vi "Frequency Response (Real-Im).vi"(0 "scaled signal X [EUx]":dbl[](array[numeric]) format="%.2f", 1 "scaled signal Y [EUy]":dbl[](array[numeric]) format="%.2f", 2 "sampling frequency [Hz]":dbl=10000.0 format="%.2f", 4 "channel X info":T2={"sensor sensitivity [mV/EU]"=1000.0, "engineering units"=1, "dB reference [EU]"=1.0, "custom label"="EU", "weighting filter"=0, "pregain [dB]"=0.0} {"pregain [dB]" format="%.2f"; "weighting filter" items=["Linear", "A-weighting", "B-weighting", "C-weighting", "ITU-R 468-4", "Dolby", "CCITT", "C-message"]; "dB reference [EU]" format="%^.1e"; "engineering units" items=["custom..."=0, "V"=1, "A"=21, "Pa"=2, "N"=20, "g"=3, "m/s^2"=4, "m/s"=5, "m"=6, "mm/s"=12, "mm"=13, "microns/s"=14, "microns"=15, "in/s^2"=7, "in/s"=8, "in"=9, "mils/s"=10, "mils"=11, "rad/s^2"=16, "rad/s"=17, "rad"=18, "strain"=19]; "sensor sensitivity [mV/EU]" format="%.2f"}, 5 "channel Y info":T2={"sensor sensitivity [mV/EU]"=1000.0, "engineering units"=1, "dB reference [EU]"=1.0, "custom label"="EU", "weighting filter"=0, "pregain [dB]"=0.0} {"pregain [dB]" format="%.2f"; "weighting filter" items=["Linear", "A-weighting", "B-weighting", "C-weighting", "ITU-R 468-4", "Dolby", "CCITT", "C-message"]; "dB reference [EU]" format="%^.1e"; "engineering units" items=["custom..."=0, "V"=1, "A"=21, "Pa"=2, "N"=20, "g"=3, "m/s^2"=4, "m/s"=5, "m"=6, "mm/s"=12, "mm"=13, "microns/s"=14, "microns"=15, "in/s^2"=7, "in/s"=8, "in"=9, "mils/s"=10, "mils"=11, "rad/s^2"=16, "rad/s"=17, "rad"=18, "strain"=19]; "sensor sensitivity [mV/EU]" format="%.2f"}, 6 "window":T6=1 items=["None"=0, "Hanning"=1, "Hamming"=2, "Blackman-Harris"=3, "Exact Blackman"=4, "Blackman"=5, "Flat Top"=6, "4 Term B-Harris "=7, "7 Term B-Harris"=8, "Low Sidelobe"=9, "Force - Exponential"=10, "Blackman Nuttall"=11, "Triangle"=30, "Bartlett-Hanning"=31, "Bohman"=32, "Parzen"=33, "Welch"=34, "Kaiser"=60, "Dolph-Chebyshev"=61, "Gaussian"=62], 7 "reset averaging (T)":bool=TRUE, 8 "force/exp settings":T5={"force window [%]"=50.0, "exponential window [%]"=10.0} {"exponential window [%]" min=0.0 max=100.0 format="%.2f"; "force window [%]" min=0.0 max=100.0 format="%.2f"}, 9 "averaging parameters":T1={"averaging mode"=enum."RMS averaging", "weighting mode"=enum."Linear", "number of averages"=10} {"number of averages" min=1}, 10 "FRF mode":enum16{"H1", "H2", "H3"}(ring)) -> (12 "df [Hz]":dbl format="%.2f", 13 "window constants":cluster{"eq noise BW":dbl, "coherent gain":dbl} {"coherent gain" format="%.2f"; "eq noise BW" format="%.2f"}, 14 "real part [EUy/EUx rms]":dbl[](array[numeric]) format="%.2f", 15 "imaginary part [EUy/EUx rms]":dbl[](array[numeric]) format="%.2f", 16 "unit label":string, 17 "coherence":dbl[](array[numeric]) format="%.2f", 18 "averages completed":dbl format="%.2f", 19 "error out":errorcluster)   [LabVIEW 2017]
doc: "Computes the frequency response and the coherence based on the input signals. Typically, X signal is the stimulus, and Y signal is the response of the system. Results are returned as real and imaginary parts.\nFrequency response is typically an averaged measurement. Each block of data corresponds to a single FFT block and must be passed individually to this VI. The first time this VI is called, reset averaging must be TRUE (default value), to start a new averaging process. For subsequent calls, reset averaging must be FALSE to continue the averaging process. Averages completed returns the number of averages completed so far.\nAveraging parameters specifies how the averaging is performed. This includes the averaging mode (no averaging, vector averaging, or RMS averaging), the weighting mode (linear or exponential), and the number of averages (used only if the weighting mode is exponential)."
uses:
  <vilib>/addons/_NISVFA/_Shared subVIs/Controls/svc_Window [Dual FFT].ctl
  <vilib>/addons/Sound and Vibration/compatibility/Controls/svl_Channel Info.ctl
  <vilib>/addons/Sound and Vibration/compatibility/Controls/svl_Engineering Units Text Ring.ctl
  <vilib>/addons/Sound and Vibration/compatibility/Controls/svl_Weighting Filter Text Ring.ctl
  <vilib>/Analysis/4window.llb/Force Window (DBL).vi
  <vilib>/Analysis/4window.llb/Exponential Window (DBL).vi
  <vilib>/Analysis/2dsp.llb/Real FFT.vi
  <vilib>/Analysis/2dsp.llb/Power Spectrum (DBL).vi
  <vilib>/Analysis/2dsp.llb/Cross Power (DBL).vi
  <vilib>/Analysis/0measdsp.llb/Scaled Time Domain Window (DBL).vi
  <vilib>/Analysis/NI_AALPro.lvlib
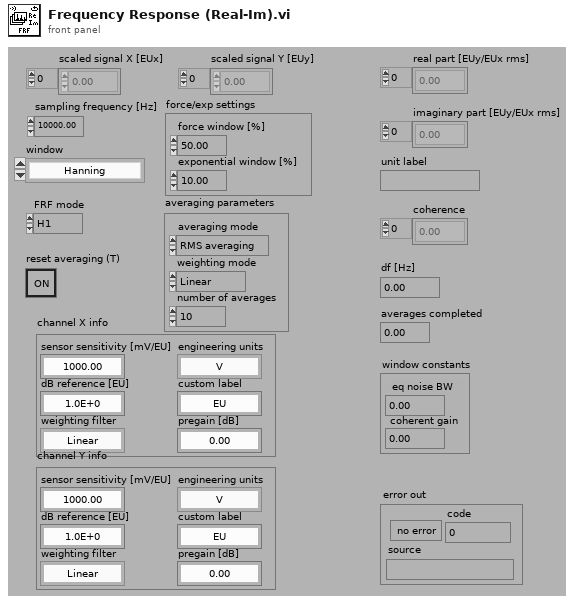
[diagram p1: front panel]
types:
  T1 = cluster{"averaging mode":enum16{"No averaging", "Vector averaging", "RMS averaging"}, "weighting mode":enum16{"Linear", "Exponential"}, "number of averages":u32}
  T2 = typedef "svl_Channel Info.ctl" = cluster{"sensor sensitivity [mV/EU]":dbl, "engineering units":T3, "dB reference [EU]":dbl, "custom label":string, "weighting filter":T4, "pregain [dB]":dbl}
  T3 = typedef "svl_Engineering Units Text Ring.ctl" = u16
  T4 = typedef "svl_Weighting Filter Text Ring.ctl" = u16
  T5 = cluster{"force window [%]":dbl, "exponential window [%]":dbl}
  T6 = typedef "svc_Window [Dual FFT].ctl" = u32
  T7 = enum16{"No averaging", "Vector averaging", "RMS averaging"}
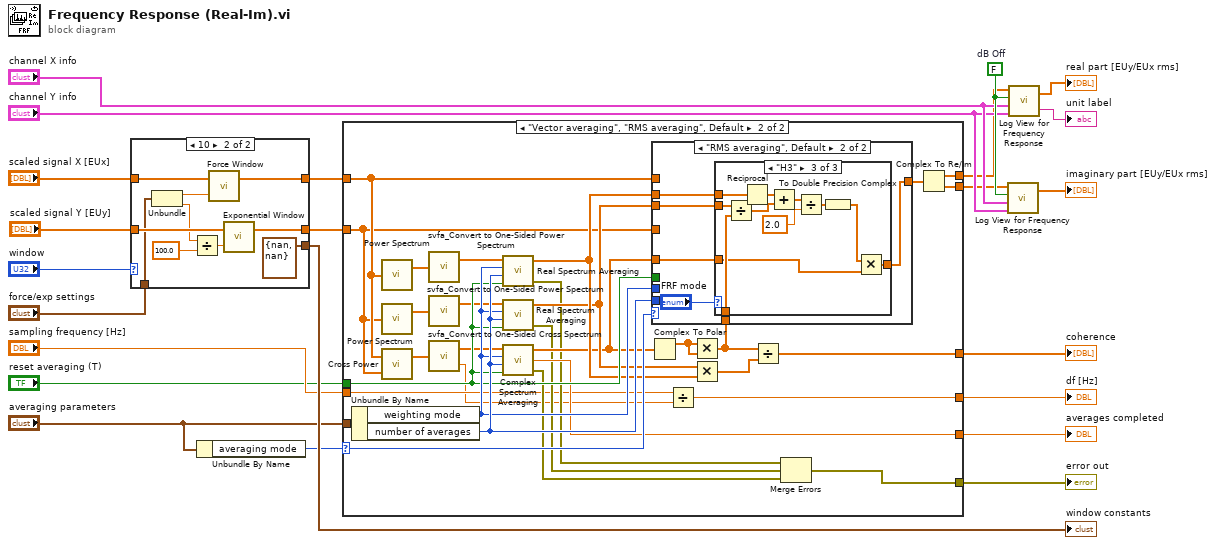
[diagram p0: block diagram]
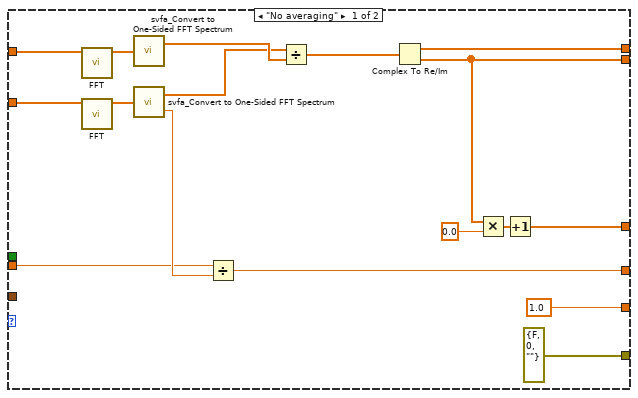
[diagram p2: hidden frame]
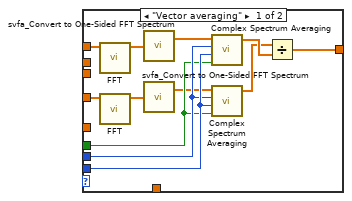
[diagram p3: hidden frame]
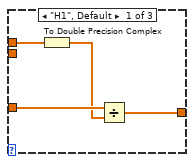
[diagram p4: hidden frame]
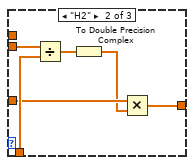
[diagram p5: hidden frame]
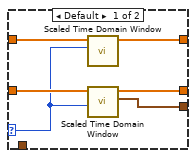
[diagram p6: hidden frame]
diagram:
  w10 = FALSE  # dB Off
  n1 = case shown="10" "window" {
    selector: "window" -> [w24 _]
    tunnel: "scaled signal X [EUx]" -> [w29 w39]
    tunnel: "scaled signal Y [EUy]" -> [w28 w38]
    tunnel: "force/exp settings" -> [_ w34]
    tunnel: [w27 w36] -> w19
    tunnel: [w26 w35] -> w18
    tunnel: [w25 cluster{"eq noise BW":dbl, "coherent gain":dbl} {"eq noise BW"=nan, "coherent gain"=nan} ("window constants")] -> w20
    frame Default {
      n2 = call-poly <vilib>:"Scaled Time Domain Window.vi"("window"=w24, "X"=w29) -> ("Windowed X"=w27:dbl[])  [unwired: 7 in, 2 out]
      n3 = call-poly <vilib>:"Scaled Time Domain Window.vi"("window"=w24, "X"=w28) -> ("window properties"=w25:cluster{"eq noise BW":dbl, "coherent gain":dbl}, "Windowed X"=w26:dbl[])  [unwired: 7 in, 1 out]
    }
    frame 10 {
      n4 = Unbundle(w34) -> ("force window [%]"=w33:dbl, "exponential window [%]"=w32:dbl)
      n5 = Divide(x=w32, y=100.0 ("x")) -> (x/y=w37:dbl)
      n6 = call-poly <vilib>:"Force Window.vi"("duty cycle(%)"=w33, "X"=w39) -> ("Windowed X"=w36:dbl[])  [unwired: 1 out]
      n7 = call-poly <vilib>:"Exponential Window.vi"("final value"=w37, "X"=w38) -> ("Windowed X"=w35:dbl[])  [unwired: 1 out]
    }
  }
  "window constants" <- w20
  n8 = Unbundle By Name("averaging parameters") -> ("averaging mode"=w14:T7)
  n9 = case shown="\"Vector averaging\", \"RMS averaging\", Default" w14 {
    selector: w14 -> [_ w85]
    tunnel: w19 -> [w51 w64]
    tunnel: "sampling frequency [Hz]" -> [w47 w62]
    tunnel: [w46 w60] -> w13
    tunnel: "reset averaging (T)" -> [_ w82]
    tunnel: "averaging parameters" -> [_ w87]
    tunnel: [1.0 ("averages completed") w78] -> w12
    tunnel: w18 -> [w50 w63]
    tunnel: [w40 w81] -> w11
    tunnel: [errorcluster {"status"=FALSE, "code"=0, "source"=""} ("error out") w71] -> w4
    tunnel: [w44 w58] -> w2
    tunnel: [w42 w57] -> w1
    frame "No averaging" {
      n10 = call-poly <vilib>:"FFT.vi"("X"=w51) -> ("FFT {X}"=w54:cdb[])  [unwired: 9 in, 1 out]
      n11 = call-poly <vilib>:"FFT.vi"("X"=w50) -> ("FFT {X}"=w53:cdb[])  [unwired: 9 in, 1 out]
      n12 = call <vilib>:"svfa_Convert to One-Sided FFT Spectrum.vi"("two-sided FFT spectrum"=w54) -> ("one-sided FFT spectrum"=w49:cdb[])  [unwired: 1 out]
      n13 = call <vilib>:"svfa_Convert to One-Sided FFT Spectrum.vi"("two-sided FFT spectrum"=w53) -> ("one-sided FFT spectrum"=w48:cdb[], "block size"=w52:dbl)
      n14 = Divide(x=w47, y=w52) -> (x/y=w46:dbl)
      n15 = Divide(x=w48, y=w49) -> (x/y=w45:cdb[])
      n16 = Complex To Re/Im(x + iy=w45) -> (x=w44:dbl[], y=w42:dbl[])
      n17 = Multiply(x=w42, y=0.0) -> (x*y=w41:dbl[])
      n18 = Increment(x=w41) -> (x+1=w40:dbl[])
    }
    frame "Vector averaging", "RMS averaging", Default {
      n19 = Unbundle By Name(w87) -> ("weighting mode"=w83:enum16{"Linear", "Exponential"}, "number of averages"=w84:u32)
      n20 = call-poly <vilib>:"Power Spectrum.vi"("X"=w64) -> ("Power Spectrum"=w69:dbl[])  [unwired: 1 out]
      n21 = call-poly <vilib>:"Power Spectrum.vi"("X"=w63) -> ("Power Spectrum"=w68:dbl[])  [unwired: 1 out]
      n22 = call-poly <vilib>:"Cross Power.vi"("Y"=w63, "X"=w64) -> ("Sxy"=w70:cdb[])  [unwired: 1 out]
      n23 = call <vilib>:"svfa_Convert to One-Sided Power Spectrum.vi"("two-sided power spectrum"=w69) -> ("one-sided power spectrum"=w67:dbl[])  [unwired: 1 out]
      n24 = call <vilib>:"svfa_Convert to One-Sided Power Spectrum.vi"("two-sided power spectrum"=w68) -> ("one-sided power spectrum"=w66:dbl[])  [unwired: 1 out]
      n25 = call <vilib>:"svfa_Convert to One-Sided Cross Spectrum.vi"("two-sided cross spectrum"=w70) -> ("one-sided cross spectrum"=w65:cdb[], "block size"=w61:dbl)
      n26 = call <vilib>:"Real Spectrum Averaging.vi"("reset averaging (T)"=w82, "number of averages"=w84, "weighting mode"=w83, "real spectrum"=w67) -> ("error out"=w74:errorcluster, "averaged real spectrum"=w80:dbl[])  [unwired: 1 out]
      n27 = call <vilib>:"Real Spectrum Averaging.vi"("reset averaging (T)"=w82, "number of averages"=w84, "weighting mode"=w83, "real spectrum"=w66) -> ("error out"=w73:errorcluster, "averaged real spectrum"=w79:dbl[])  [unwired: 1 out]
      n28 = call <vilib>:"Complex Spectrum Averaging.vi"("reset averaging (T)"=w82, "number of averages"=w84, "weighting mode"=w83, "complex spectrum"=w65) -> ("error out"=w72:errorcluster, "averages completed"=w78:dbl, "averaged complex spectrum"=w76:cdb[])
      n29 = Complex To Polar(r * e^(i*theta)=w76) -> (r=w77:dbl[])  [unwired: 1 out]
      n30 = Divide(x=w62, y=w61) -> (x/y=w60:dbl)
      n31 = Multiply(x=w77, y=w77) -> (x*y=w75:dbl[])
      n32 = case shown="\"RMS averaging\", Default" w85 {
        tunnel: w64 -> [w90 _]
        tunnel: w63 -> [w91 _]
        tunnel: w84 -> [w97 _]
        tunnel: w83 -> [w96 _]
        tunnel: w82 -> [w95 _]
        tunnel: w76 -> [_ w101]
        tunnel: w80 -> [_ w104]
        tunnel: w79 -> [_ w103]
        tunnel: w75 -> [_ w102]
        tunnel: [w94 w100] -> w59
        frame "Vector averaging" {
          n33 = call-poly <vilib>:"FFT.vi"("X"=w90) -> ("FFT {X}"=w93:cdb[])  [unwired: 9 in, 1 out]
          n34 = call-poly <vilib>:"FFT.vi"("X"=w91) -> ("FFT {X}"=w92:cdb[])  [unwired: 9 in, 1 out]
          n35 = call <vilib>:"svfa_Convert to One-Sided FFT Spectrum.vi"("two-sided FFT spectrum"=w93) -> ("one-sided FFT spectrum"=w89:cdb[])  [unwired: 1 out]
          n36 = call <vilib>:"svfa_Convert to One-Sided FFT Spectrum.vi"("two-sided FFT spectrum"=w92) -> ("one-sided FFT spectrum"=w88:cdb[])  [unwired: 1 out]
          n37 = call <vilib>:"Complex Spectrum Averaging.vi"("reset averaging (T)"=w95, "number of averages"=w97, "weighting mode"=w96, "complex spectrum"=w89) -> ("averaged complex spectrum"=w99:cdb[])  [unwired: 2 out]
          n38 = call <vilib>:"Complex Spectrum Averaging.vi"("reset averaging (T)"=w95, "number of averages"=w97, "weighting mode"=w96, "complex spectrum"=w88) -> ("averaged complex spectrum"=w98:cdb[])  [unwired: 2 out]
          n39 = Divide(x=w98, y=w99) -> (x/y=w94:cdb[])
        }
        frame "RMS averaging", Default {
          n40 = case shown="\"H3\"" "FRF mode" {
            tunnel: w104 -> [w109 _ w126]
            tunnel: w103 -> [_ w115 w125]
            tunnel: w102 -> [_ w114 w124]
            tunnel: w101 -> [w107 w112 w118]
            tunnel: [w108 w111 w119] -> w100
            frame "H1", Default {
              n41 = To Double Precision Complex(1:w109) -> (0:w106:cdb[])
              n42 = Divide(x=w107, y=w106) -> (x/y=w108:cdb[])
            }
            frame "H2" {
              n43 = Divide(x=w115, y=w114) -> (x/y=w113:dbl[])
              n44 = To Double Precision Complex(1:w113) -> (0:w110:cdb[])
              n45 = Multiply(x=w112, y=w110) -> (x*y=w111:cdb[])
            }
            frame "H3" {
              n46 = Divide(x=w125, y=w124) -> (x/y=w122:dbl[])
              n47 = Reciprocal(x=w126) -> (1/x=w123:dbl[])
              n48 = Add(x=w123, y=w122) -> (x+y=w121:dbl[])
              n49 = Divide(x=w121, y=2.0) -> (x/y=w117:dbl[])
              n50 = To Double Precision Complex(1:w117) -> (0:w116:cdb[])
              n51 = Multiply(x=w116, y=w118) -> (x*y=w119:cdb[])
            }
          }
        }
      }
      n52 = Multiply(x=w79, y=w80) -> (x*y=w86:dbl[])
      n53 = Divide(x=w75, y=w86) -> (x/y=w81:dbl[])
      n54 = Merge Errors(w74, w73, w72) -> (w71:errorcluster)
      n55 = Complex To Re/Im(x + iy=w59) -> (x=w58:dbl[], y=w57:dbl[])
    }
  }
  "df [Hz]" <- w13
  "averages completed" <- w12
  "coherence" <- w11
  "error out" <- w4
  n56 = call <vilib>:"Log View for Frequency Response.vi"("channel Y info"="channel Y info", "channel X info"="channel X info", "dB On (T)"=w10, "FRF [EUy/EUx]"=w1) -> ("log view FRF [dB EUy/EUx]"=→"imaginary part [EUy/EUx rms]":dbl[])  [unwired: 1 out]
  n57 = call <vilib>:"Log View for Frequency Response.vi"("channel Y info"="channel Y info", "channel X info"="channel X info", "dB On (T)"=w10, "FRF [EUy/EUx]"=w2) -> ("unit label"=→"unit label":string, "log view FRF [dB EUy/EUx]"=→"real part [EUy/EUx rms]":dbl[])
